vi "DOC-HTML-state-machine.vi"(6 "header":string, 7 "VI paths":path[](array[path]), 8 "error in":errorcluster, 9 "HTML":string[](array[string]), 10 "states":T1[](array[typedef]), 11 "report file destination":path) -> (0 "error out":errorcluster)   [LabVIEW 2014]
uses:
  controls/state-machine.ctl
  <vilib>/printing/ReportDocExtensions.llb/Append Front Panel Image to Report (path).vi
  <vilib>/printing/ReportDocExtensions.llb/Append VI Block Diagram to Report (path).vi
  <vilib>/printing/ReportDocExtensions.llb/Append VI Icon to Report (path).vi
  <vilib>/printing/ReportDocExtensions.llb/Append VI Description to Report (path).vi
  <vilib>/printing/ReportDocExtensions.llb/Append VI Hierarchy to Report (path).vi
  <vilib>/printing/ReportDocExtensions.llb/Append VI List of SubVIs to Report (path).vi
  <vilib>/printing/OpenHTMLReport.llb/Open HTML Report in Browser (Refnum).vi
  <vilib>/printing/ReportDocExtensions.llb/Append VI History to Report (path).vi
  <vilib>/Utility/NIReport.llb/NI_report.lvclass
  <vilib>/Utility/NIReport.llb/NI_ReportGenerationCore.lvlib
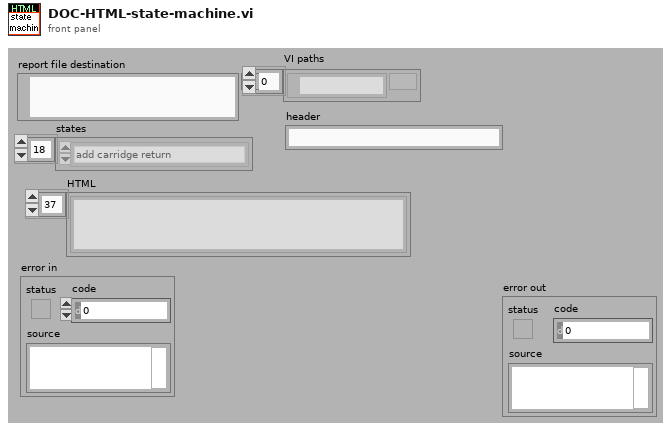
[diagram p1: front panel]
types:
  T1 = typedef "state-machine.ctl" = enum16{"add carridge return", "init", "Read-inputs", "edit generated file", "end", "Add front panel", "Add Block Diagram", "Add VI icon", "Add VI description", "Add VI hiearchy", "Add list of sub vis", "add custom html", "open report in browser", "Save report to file", "dispose report", "Add header text", "Create style .css", "add-red-box-header", "Delete Temp Files", "Remove-path-element", "add-revision-history", "add-icon-image-only"}
  T2 = enum16{"Standard Report", "HTML", "Word", "Excel"}
  T3 = enum16{"open", "replace", "create", "open or create", "replace or create", "replace or create with confirmation"}
  T4 = cluster{"report out":refnum<class "NI_report.lvclass">, "VI paths":path[], "report file destination":path, "number of lines":i32, "image format (PNG)":enum32{"PNG", "JPEG", "GIF"}}
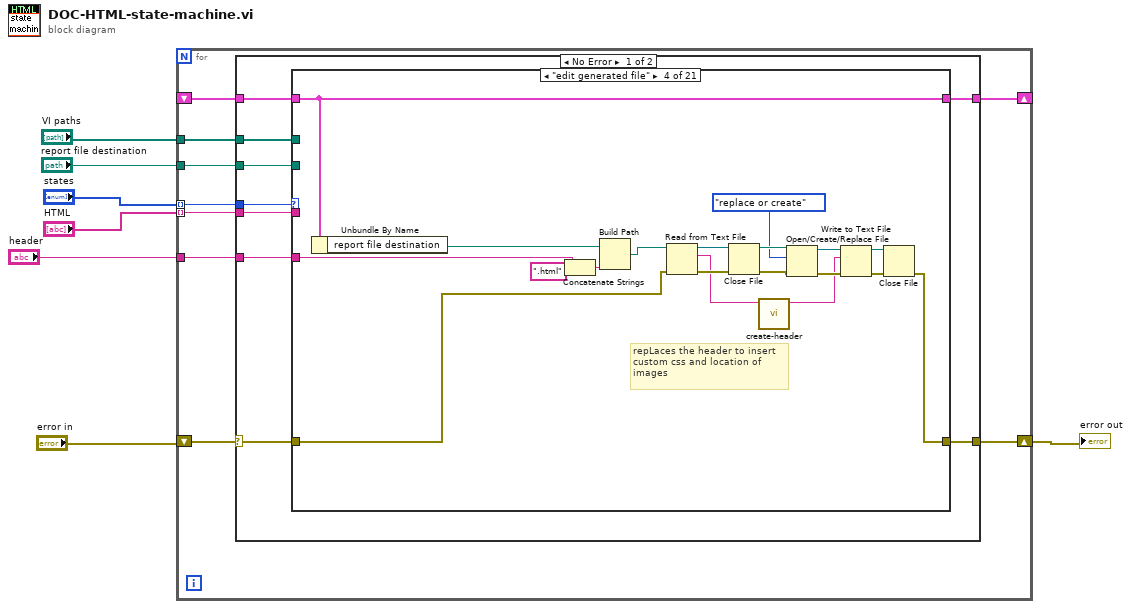
[diagram p0: block diagram]
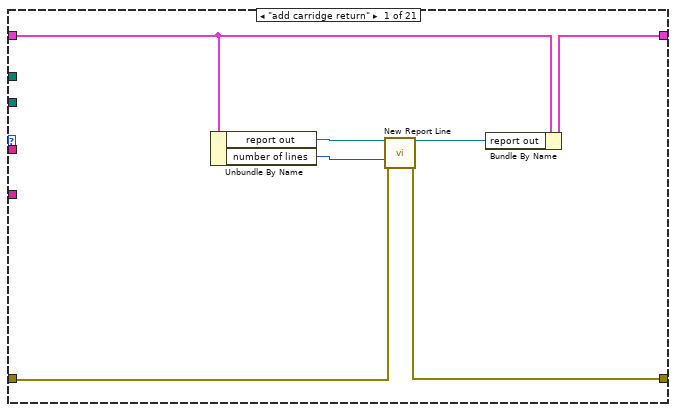
[diagram p2: hidden frame]
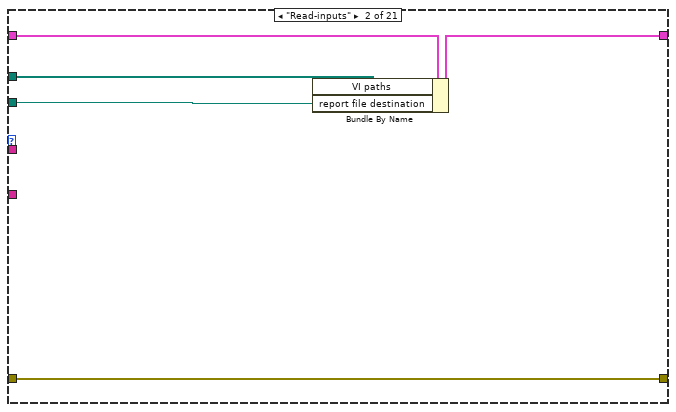
[diagram p3: hidden frame]
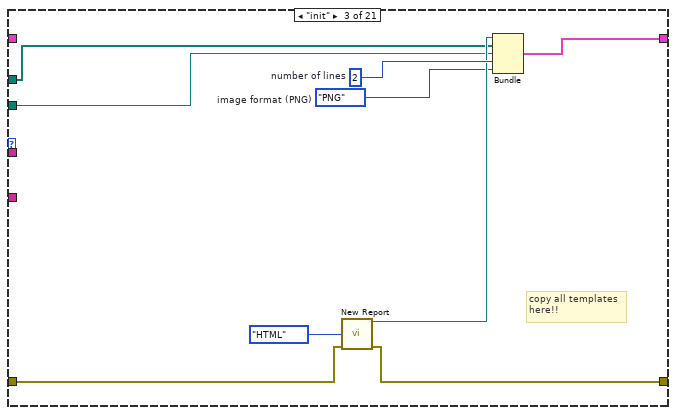
[diagram p4: hidden frame]
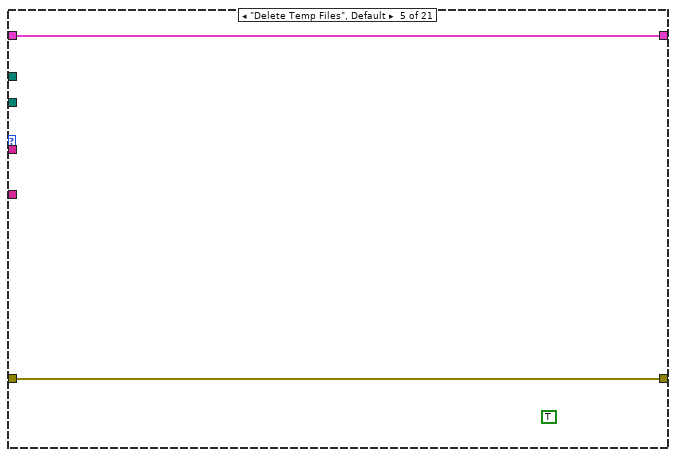
[diagram p5: hidden frame]
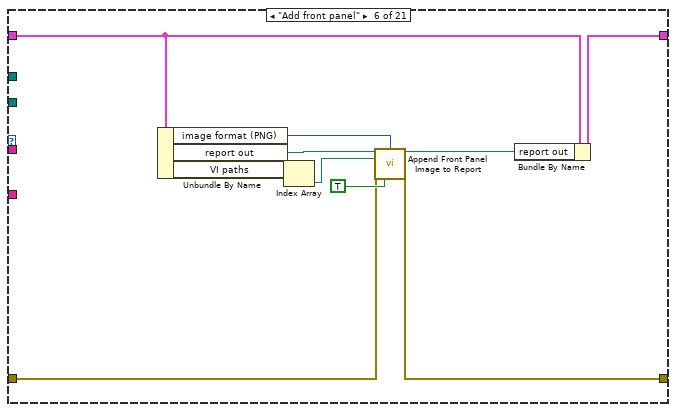
[diagram p6: hidden frame]
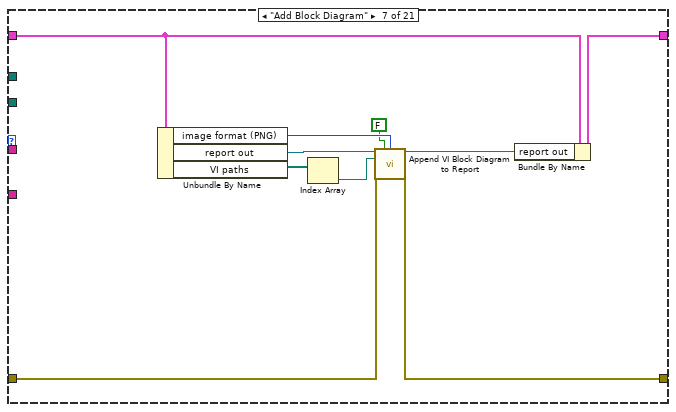
[diagram p7: hidden frame]
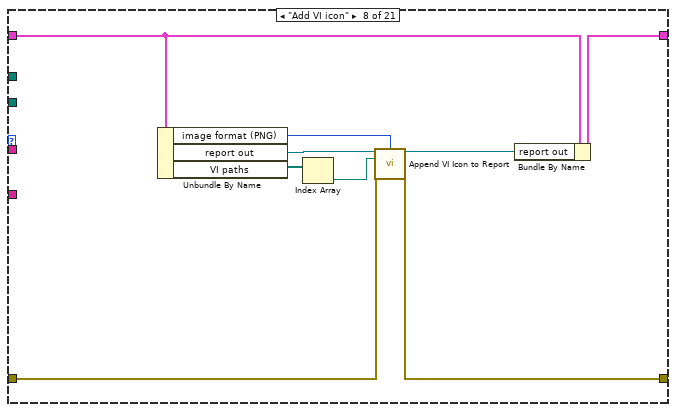
[diagram p8: hidden frame]
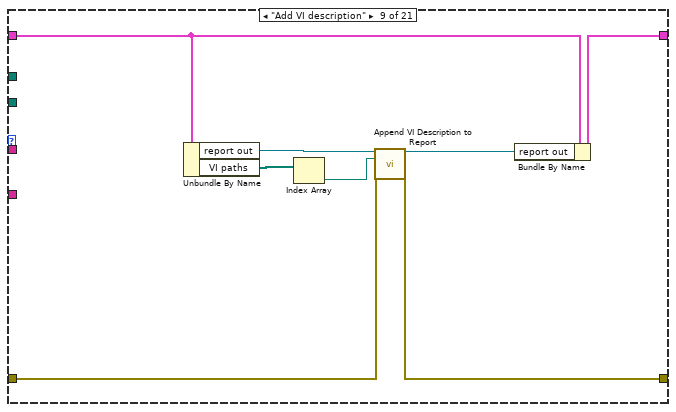
[diagram p9: hidden frame]
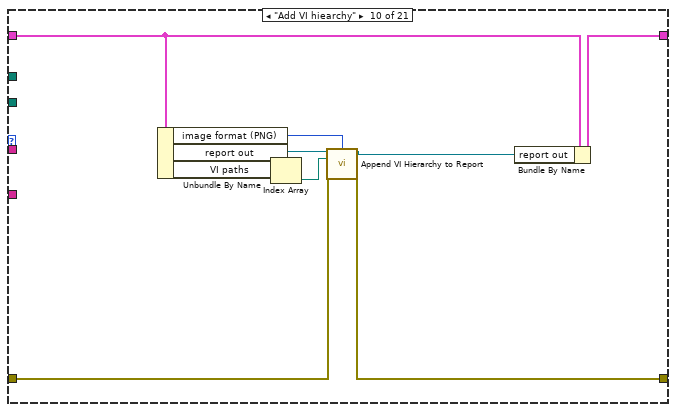
[diagram p10: hidden frame]
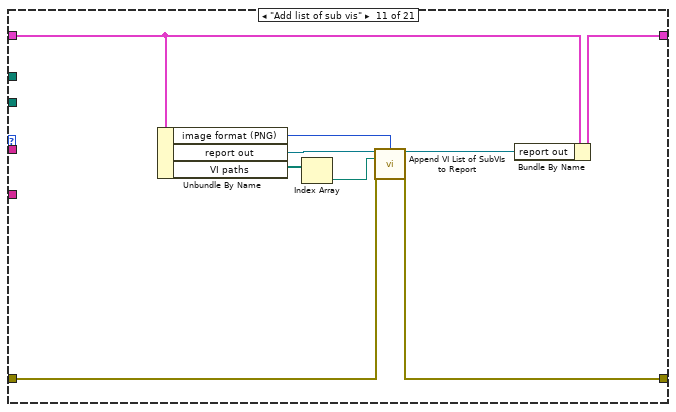
[diagram p11: hidden frame]
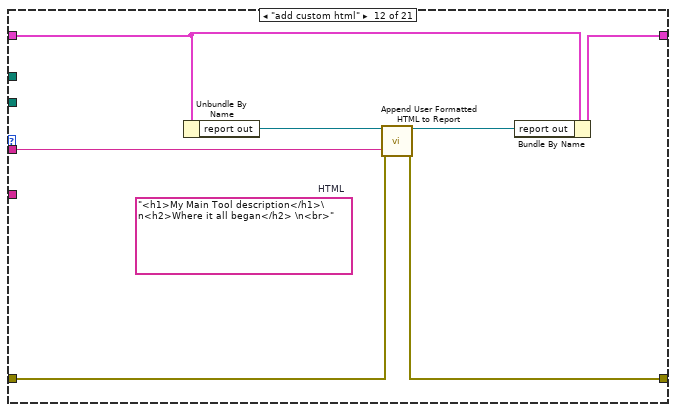
[diagram p12: hidden frame]
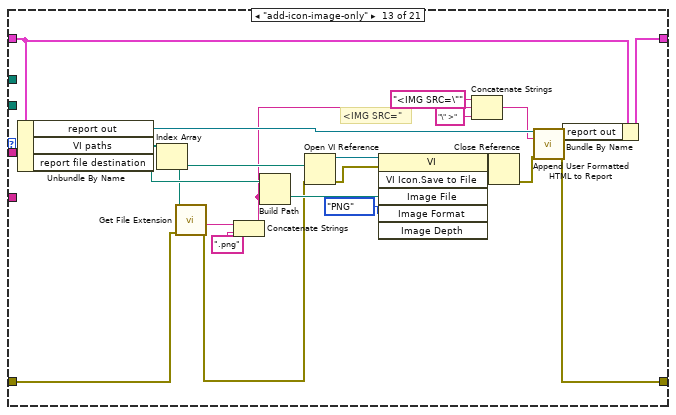
[diagram p13: hidden frame]
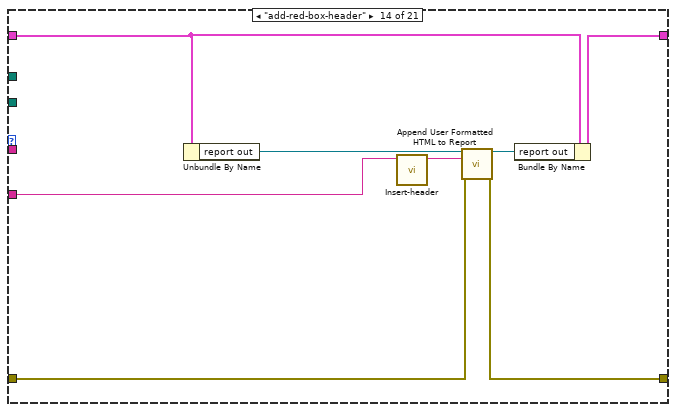
[diagram p14: hidden frame]
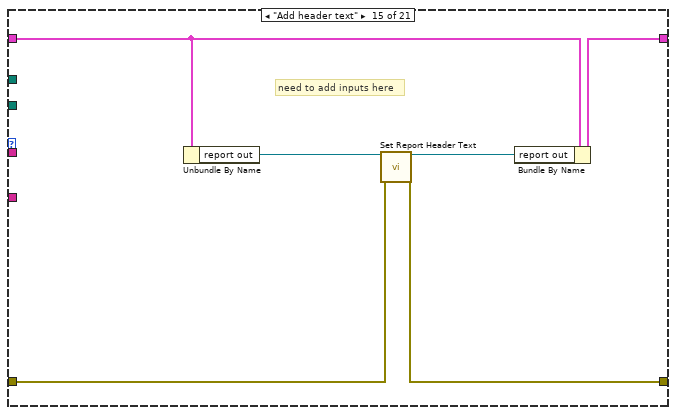
[diagram p15: hidden frame]
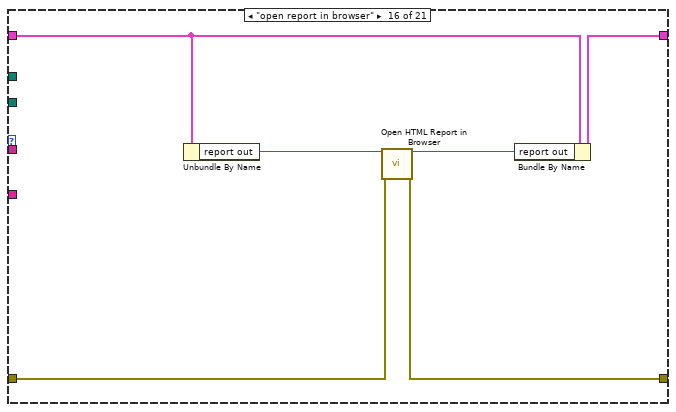
[diagram p16: hidden frame]
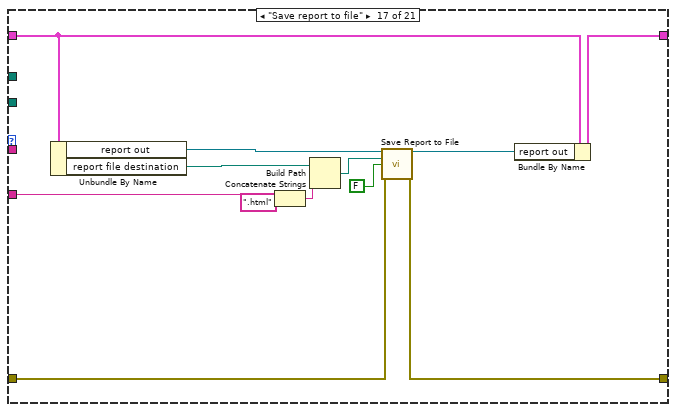
[diagram p17: hidden frame]
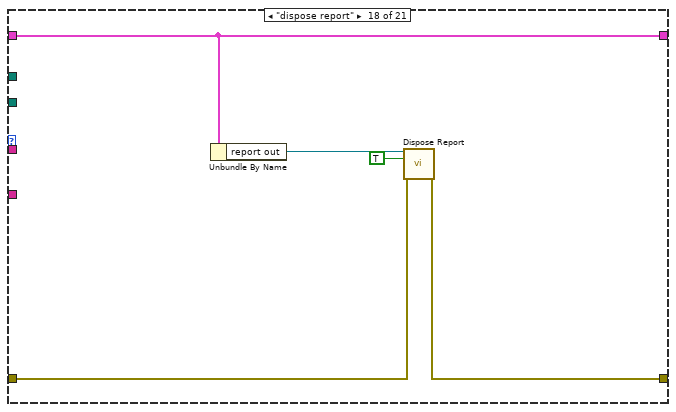
[diagram p18: hidden frame]
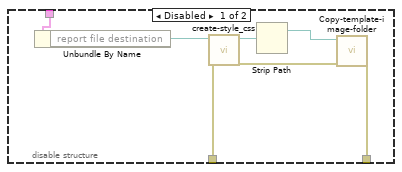
[diagram p20: hidden frame]
diagram:
  n1 = for {
    tunnel: "states" -> [w12] mode=indexing
    shift-right: [w16] -> _
    shift-left: _ -> [w15]
    shift-right: [w14] -> w3
    shift-left: "error in" -> [w13]
    tunnel: "HTML" -> [w11] mode=indexing
    tunnel: "report file destination" -> [w10]
    tunnel: "VI paths" -> [w9]
    tunnel: "header" -> [w8]
    n2 = case shown="No Error" w13 {
      selector: w13 -> [w22 w215]
      tunnel: [w25 w215] -> w14
      tunnel: [w24 w216] -> w16
      tunnel: w15 -> [w23 w216]
      tunnel: w12 -> [w21 _]
      tunnel: w11 -> [w20 _]
      tunnel: w10 -> [w19 _]
      tunnel: w9 -> [w18 _]
      tunnel: w8 -> [w17 _]
      frame No Error {
        n3 = case shown="\"edit generated file\"" w21 {
          tunnel: [w26 w33 w41 w55 w66 w71 w83 w91 w99 w109 w117 w125 w148 w156 w162 w168 w180 w187 w190 w207 w208] -> w25
          tunnel: [w30 w35 w45 w65 w67 w74 w85 w94 w102 w111 w120 w128 w151 w159 w165 w171 w183 w186 w192 w203 w212] -> w24
          tunnel: w23 -> [w31 w36 _ w65 w67 w75 w86 w95 w103 w112 w121 w129 w152 w160 w166 w172 w184 w186 w192 w204 w213]
          tunnel: w22 -> [w28 w33 w44 w48 w66 w72 w84 w92 w100 w110 w118 w124 w135 w155 w161 w167 w179 w188 w191 w207 w208]
          tunnel: w20 -> [_ _ _ _ _ _ _ _ _ _ _ w123 _ _ _ _ _ _ _ _ _]
          tunnel: w19 -> [_ w34 w40 _ _ _ _ _ _ _ _ _ _ _ _ _ _ _ _ _ _]
          tunnel: w18 -> [_ w37 w39 _ _ _ _ _ _ _ _ _ _ _ _ _ _ _ _ _ _]
          tunnel: w17 -> [_ _ _ w47 _ _ _ _ _ _ _ _ _ w153 _ _ w173 _ _ _ _]
          frame "add carridge return" {
            n4 = Unbundle By Name(w31) -> ("report out"=w32:refnum<class "NI_report.lvclass">, "number of lines"=w27:i32)
            n5 = call-dynamic "New Report Line.vi"("report in"=w32, "number of lines (1)"=w27, "error in (no error)"=w28) -> ("report out"=w29:refnum<class "NI_report.lvclass">, "error out"=w26:errorcluster)  [unwired: 11 out]
            n6 = Bundle By Name(cluster=w31, "report out"=w29) -> (w30:T4)
          }
          frame "Read-inputs" {
            n7 = Bundle By Name(cluster=w36, "VI paths"=w37, "report file destination"=w34) -> (w35:T4)
          }
          frame "init" {
            w38 = enum32{"PNG", "JPEG", "GIF"}."PNG"  # image format (PNG)
            w43 = 2  # number of lines
            # "copy all templates\nhere!!"
            n8 = call <vilib>:"New Report.vi"("report type"=T2."HTML", "error in (no error)"=w44) -> ("report out"=w42:refnum<class "NI_report.lvclass">, "error out"=w41:errorcluster)  [unwired: 4 in, 8 out]
            n9 = Bundle("report out"=w42, "VI paths"=w39, "report file destination"=w40, "number of lines"=w43, "image format (PNG)"=w38) -> (w45:T4)  [unwired: 1 out]
          }
          frame "edit generated file" {
            # "repLaces the header to insert \ncustom css and location of\nimages"
            n10 = Unbundle By Name(w65) -> ("report file destination"=w52:path)
            n11 = Concatenate Strings(w47, ".html" ("string")) -> (w51:string)
            n12 = Build Path(base path=w52, name or relative path=w51) -> (appended path=w49:path)
            n13 = Read from Text File(file (use dialog)=w49, error in=w48) -> (refnum out=w64:refnum<file>, text=w54:string, error out=w60:errorcluster)  [unwired: 3 out]
            n14 = Close File(refnum=w64, error in=w60) -> (path=w63:path, error out=w59:errorcluster)
            n15 = call "create-header.vi"("htmlin"=w54) -> ("replaced header"=w53:string)  [unwired: 10 out]
            n16 = Open/Create/Replace File(file path (use dialog)=w63, error in=w59, operation (0:open)=T3."replace or create") -> (refnum out=w62:refnum<file>, error out=w58:errorcluster)  [unwired: 4 out]
            n17 = Write to Text File(file (use dialog)=w62, text=w53, error in=w58) -> (refnum out=w61:refnum<file>, error out=w57:errorcluster)  [unwired: 2 out]
            n18 = Close File(refnum=w61, error in=w57) -> (error out=w55:errorcluster)  [unwired: 1 out]
          }
          frame "Delete Temp Files", Default {
            (unwired) TRUE
          }
          frame "Add front panel" {
            n19 = Unbundle By Name(w75) -> ("image format (PNG)"=w68:enum32{"PNG", "JPEG", "GIF"}, "report out"=w76:refnum<class "NI_report.lvclass">, "VI paths"=w69:path[])
            n20 = Index Array(array=w69) -> (element=w70:path)  [unwired: 1 in]
            n21 = call-poly <vilib>:"Append Front Panel Image to Report.vi"("report in"=w76, "image format (jpeg)"=w68, "VI"=w70, "error in (no error)"=w72, "visible area only?"=TRUE) -> ("report out"=w73:refnum<class "NI_report.lvclass">, "error out"=w71:errorcluster)  [unwired: 3 in, 6 out]
            n22 = Bundle By Name(cluster=w75, "report out"=w73) -> (w74:T4)
          }
          frame "Add Block Diagram" {
            n23 = Unbundle By Name(w86) -> ("image format (PNG)"=w79:enum32{"PNG", "JPEG", "GIF"}, "report out"=w87:refnum<class "NI_report.lvclass">, "VI paths"=w82:path[])
            n24 = Index Array(array=w82) -> (element=w80:path)  [unwired: 1 in]
            n25 = call-poly <vilib>:"Append VI Block Diagram to Report.vi"("report in"=w87, "hidden frames"=FALSE, "image format (jpeg)"=w79, "VI"=w80, "error in (no error)"=w84) -> ("report out"=w81:refnum<class "NI_report.lvclass">, "error out"=w83:errorcluster)  [unwired: 3 in, 6 out]
            n26 = Bundle By Name(cluster=w86, "report out"=w81) -> (w85:T4)
          }
          frame "Add VI icon" {
            n27 = Unbundle By Name(w95) -> ("image format (PNG)"=w88:enum32{"PNG", "JPEG", "GIF"}, "report out"=w96:refnum<class "NI_report.lvclass">, "VI paths"=w90:path[])
            n28 = Index Array(array=w90) -> (element=w89:path)  [unwired: 1 in]
            n29 = call-poly <vilib>:"Append VI Icon to Report.vi"("report in"=w96, "image format (jpeg)"=w88, "VI"=w89, "error in (no error)"=w92) -> ("report out"=w93:refnum<class "NI_report.lvclass">, "error out"=w91:errorcluster)  [unwired: 3 in, 7 out]
            n30 = Bundle By Name(cluster=w95, "report out"=w93) -> (w94:T4)
          }
          frame "Add VI description" {
            n31 = Unbundle By Name(w103) -> ("report out"=w104:refnum<class "NI_report.lvclass">, "VI paths"=w97:path[])
            n32 = Index Array(array=w97) -> (element=w98:path)  [unwired: 1 in]
            n33 = call-poly <vilib>:"Append VI Description to Report.vi"("report in"=w104, "VI"=w98, "error in (no error)"=w100) -> ("report out"=w101:refnum<class "NI_report.lvclass">, "error out"=w99:errorcluster)  [unwired: 1 in, 10 out]
            n34 = Bundle By Name(cluster=w103, "report out"=w101) -> (w102:T4)
          }
          frame "Add VI hiearchy" {
            n35 = Unbundle By Name(w112) -> ("image format (PNG)"=w105:enum32{"PNG", "JPEG", "GIF"}, "report out"=w113:refnum<class "NI_report.lvclass">, "VI paths"=w108:path[])
            n36 = Index Array(array=w108) -> (element=w107:path)  [unwired: 1 in]
            n37 = call-poly <vilib>:"Append VI Hierarchy to Report.vi"("report in"=w113, "image format (jpeg)"=w105, "VI"=w107, "error in (no error)"=w110) -> ("report out"=w106:refnum<class "NI_report.lvclass">, "error out"=w109:errorcluster)  [unwired: 2 in, 8 out]
            n38 = Bundle By Name(cluster=w112, "report out"=w106) -> (w111:T4)
          }
          frame "Add list of sub vis" {
            n39 = Unbundle By Name(w121) -> ("image format (PNG)"=w114:enum32{"PNG", "JPEG", "GIF"}, "report out"=w122:refnum<class "NI_report.lvclass">, "VI paths"=w116:path[])
            n40 = Index Array(array=w116) -> (element=w115:path)  [unwired: 1 in]
            n41 = call-poly <vilib>:"Append VI List of SubVIs to Report.vi"("report in"=w122, "image format (jpeg)"=w114, "VI"=w115, "error in (no error)"=w118) -> ("report out"=w119:refnum<class "NI_report.lvclass">, "error out"=w117:errorcluster)  [unwired: 3 in, 7 out]
            n42 = Bundle By Name(cluster=w121, "report out"=w119) -> (w120:T4)
          }
          frame "add custom html" {
            (unwired) "<h1>My Main Tool description</h1>\n<h2>Where it all began</h2> \n<br>"  # HTML
            n43 = Unbundle By Name(w129) -> ("report out"=w127:refnum<class "NI_report.lvclass">)
            n44 = call-dynamic "Append User Formatted HTML to Report.vi"("report in"=w127, "HTML text"=w123, "error in (no error)"=w124) -> ("report out"=w126:refnum<class "NI_report.lvclass">, "error out"=w125:errorcluster)  [unwired: 11 out]
            n45 = Bundle By Name(cluster=w129, "report out"=w126) -> (w128:T4)
          }
          frame "add-icon-image-only" {
            # "<IMG SRC=\""
            n46 = Unbundle By Name(w152) -> ("report out"=w150:refnum<class "NI_report.lvclass">, "VI paths"=w144:path[], "report file destination"=w143:path)
            n47 = Index Array(array=w144) -> (element=w138:path)  [unwired: 1 in]
            n48 = call <vilib>:"Get File Extension.vi"("error in (no error)"=w135, "file"=w138) -> ("error out"=w134:errorcluster, "filename without extension"=w137:string)  [unwired: 8 out]
            n49 = Concatenate Strings(w137, ".png" ("string")) -> (w131:string)
            n50 = Build Path(base path=w143, name or relative path=w131) -> (appended path=w142:path)
            n51 = Open VI Reference(vi path=w138, error in (no error)=w134) -> (vi reference=w147:refnum<vi>, error out=w145:errorcluster)  [unwired: 4 out]
            n52 = invoke class="VI" method="VI Icon.Save to File"(reference=w147, error in=w145, "Image File"=w142, "Image Format"=enum32{"PNG", "JPEG", "GIF", "BMP"}."PNG") -> (reference out=w146:refnum<vi>, error out=w140:errorcluster)  [unwired: 2 in, 4 out]
            n53 = Concatenate Strings("<IMG SRC=\"" ("string"), w131, "\" >" ("string")) -> (w130:string)
            n54 = Close Reference(reference=w146, error in (no error)=w140) -> (error out=w139:errorcluster)
            n55 = call-dynamic "Append User Formatted HTML to Report.vi"("report in"=w150, "HTML text"=w130, "error in (no error)"=w139) -> ("report out"=w149:refnum<class "NI_report.lvclass">, "error out"=w148:errorcluster)  [unwired: 11 out]
            n56 = Bundle By Name(cluster=w152, "report out"=w149) -> (w151:T4)
          }
          frame "add-red-box-header" {
            n57 = Unbundle By Name(w160) -> ("report out"=w158:refnum<class "NI_report.lvclass">)
            n58 = call "Insert-header.vi"("Header 1"=w153) -> ("concatenated string"=w154:string)  [unwired: 1 in, 9 out]
            n59 = call-dynamic "Append User Formatted HTML to Report.vi"("report in"=w158, "HTML text"=w154, "error in (no error)"=w155) -> ("report out"=w157:refnum<class "NI_report.lvclass">, "error out"=w156:errorcluster)  [unwired: 11 out]
            n60 = Bundle By Name(cluster=w160, "report out"=w157) -> (w159:T4)
          }
          frame "Add header text" {
            # "need to add inputs here"
            n61 = Unbundle By Name(w166) -> ("report out"=w164:refnum<class "NI_report.lvclass">)
            n62 = call-dynamic "Set Report Header Text.vi"("report in"=w164, "error in (no error)"=w161) -> ("report out"=w163:refnum<class "NI_report.lvclass">, "error out"=w162:errorcluster)  [unwired: 5 in, 7 out]
            n63 = Bundle By Name(cluster=w166, "report out"=w163) -> (w165:T4)
          }
          frame "open report in browser" {
            n64 = Unbundle By Name(w172) -> ("report out"=w170:refnum<class "NI_report.lvclass">)
            n65 = call-poly <vilib>:"Open HTML Report in Browser.vi"("report in"=w170, "error in (no error)"=w167) -> ("report out"=w169:refnum<class "NI_report.lvclass">, "error out"=w168:errorcluster)  [unwired: 1 in, 11 out]
            n66 = Bundle By Name(cluster=w172, "report out"=w169) -> (w171:T4)
          }
          frame "Save report to file" {
            n67 = Unbundle By Name(w184) -> ("report out"=w182:refnum<class "NI_report.lvclass">, "report file destination"=w175:path)
            n68 = Concatenate Strings(w173, ".html" ("string")) -> (w177:string)
            n69 = Build Path(base path=w175, name or relative path=w177) -> (appended path=w174:path)
            n70 = call-dynamic "Save Report to File.vi"("report in"=w182, "report file path"=w174, "prompt to replace? (F)"=FALSE, "error in (no error)"=w179) -> ("report out"=w181:refnum<class "NI_report.lvclass">, "error out"=w180:errorcluster)  [unwired: 1 in, 9 out]
            n71 = Bundle By Name(cluster=w184, "report out"=w181) -> (w183:T4)
          }
          frame "dispose report" {
            n72 = Unbundle By Name(w186) -> ("report out"=w189:refnum<class "NI_report.lvclass">)
            n73 = call-dynamic "Dispose Report.vi"("report in"=w189, "wait until printing completed? (T)"=TRUE, "error in (no error)"=w188) -> ("error out"=w187:errorcluster)  [unwired: 2 in, 10 out]
          }
          frame "Create style .css" {
            # "generates a cascading style sheet for the web page and copies the\nneeded images and its foler"
            n74 = disable-structure shown="Enabled" {
              disable-tunnel: w192 -> [w199 _]
              disable-tunnel: w191 -> [w197 w200]
              disable-tunnel: [w193 w200] -> w190
              frame Disabled {
                n75 = Unbundle By Name(w199) -> ("report file destination"=w198:path)
                n76 = call "create-style_css.vi"("error in (no error)"=w197, "path to .css file"=w198) -> ("error out"=w194:errorcluster, "path"=w196:path)  [unwired: 8 out]
                n77 = Strip Path(path=w196) -> (stripped path=w195:path)  [unwired: 1 out]
                n78 = call "Copy-template-image-folder.vi"("error in"=w194, "target path (use dialog)"=w195) -> ("error out"=w193:errorcluster)  [unwired: 9 out]
              }
              frame Enabled {
              }
            }
          }
          frame "Remove-path-element" {
            n79 = Unbundle By Name(w204) -> ("VI paths"=w206:path[])
            n80 = Delete From Array(array=w206, length=1, index=0) -> (array with subset deleted=w205:path[])  [unwired: 1 out]
            n81 = Bundle By Name(cluster=w204, "VI paths"=w205) -> (w203:T4)
          }
          frame "add-revision-history" {
            n82 = Unbundle By Name(w213) -> ("report out"=w211:refnum<class "NI_report.lvclass">, "VI paths"=w214:path[])
            n83 = Index Array(array=w214) -> (element=w209:path)  [unwired: 1 in]
            n84 = call-poly <vilib>:"Append VI History to Report.vi"("report in"=w211, "VI"=w209) -> ("report out"=w210:refnum<class "NI_report.lvclass">)  [unwired: 2 in, 11 out]
            n85 = Bundle By Name(cluster=w213, "report out"=w210) -> (w212:T4)
          }
        }
      }
      frame Error {
      }
    }
  }
  "error out" <- w3
